vi "RF Sweep.vi"() -> ()   [LabVIEW 2012]
uses:
  <vilib>/DAQmx/read.llb/DAQmx Read (Counter U32 1Chan 1Samp).vi
  <vilib>/Utility/file.llb/Write To Spreadsheet File (DBL).vi
  <vilib>/DAQmx/miscellaneous.llb/DAQmx Fill In Error Info.vi
  <vilib>/DAQmx/create/channels.llb/DAQmx Create Channel (CO-Pulse Generation-Ticks).vi
  <vilib>/DAQmx/configure/timing.llb/DAQmx Timing (Implicit).vi
  <vilib>/DAQmx/create/channels.llb/DAQmx Create Channel (CI-Count Edges).vi
  <vilib>/DAQmx/configure/timing.llb/DAQmx Timing (Sample Clock).vi
  <resource>/objmgr/daqmx.rc
panel:
  in  "Time Target (s)":dbl=1.0
  out "freq":dbl
  out "diff":dbl
  out "loop":i32
  in  "file path (dialog if empty)":path
  out "Z Position 2":dbl
  out "Y Position 2":dbl
  out "X Position 2":dbl
  in  "CW for tracking":bool
  in  "Y Parameters":T1={"Number of Y Steps"=200, "Max Y (V)"=2.0, "Min Y (V)"=-2.0}
  in  "X":T2={"Number of X Steps"=200, "Max X (V)"=2.0, "Min X (V)"=-2.0}
  in  "Z Position":dbl
  in  "Y Position":dbl
  in  "X Position":dbl
  in  "Z-track?":bool
  out "XY Graph":cluster{"Y":dbl[], "Y":dbl[]}[](graph)
  in  "Freq Max":dbl=485493835.2340852
  in  "Freq  Step":dbl=485493835.2340852
  in  "Freq Min":dbl=485493835.2340852
  in  "power":dbl
  in  "Measure N Loops":i32
  in  "stop":bool
  out "no pi":u32
  out "pi":u32
  in  "Path to spinapi.dll":path=path "C:/SpinCore/SpinAPI/dll/spinapi64.dll"
  in  "Pulse offset":dbl
  in  "Tau":dbl
  in  "RF Pulse":dbl
  in  "Rabi Freq":dbl
  in  "MW Delay":dbl
  in  "APD signal width":dbl=5e-07
  in  "Signal Delay":dbl=6e-07
  in  "AOM Rest time":dbl=1e-06
  in  "AOM Pulse length":dbl=2.5e-06
  in  "N Loop":i32=10000
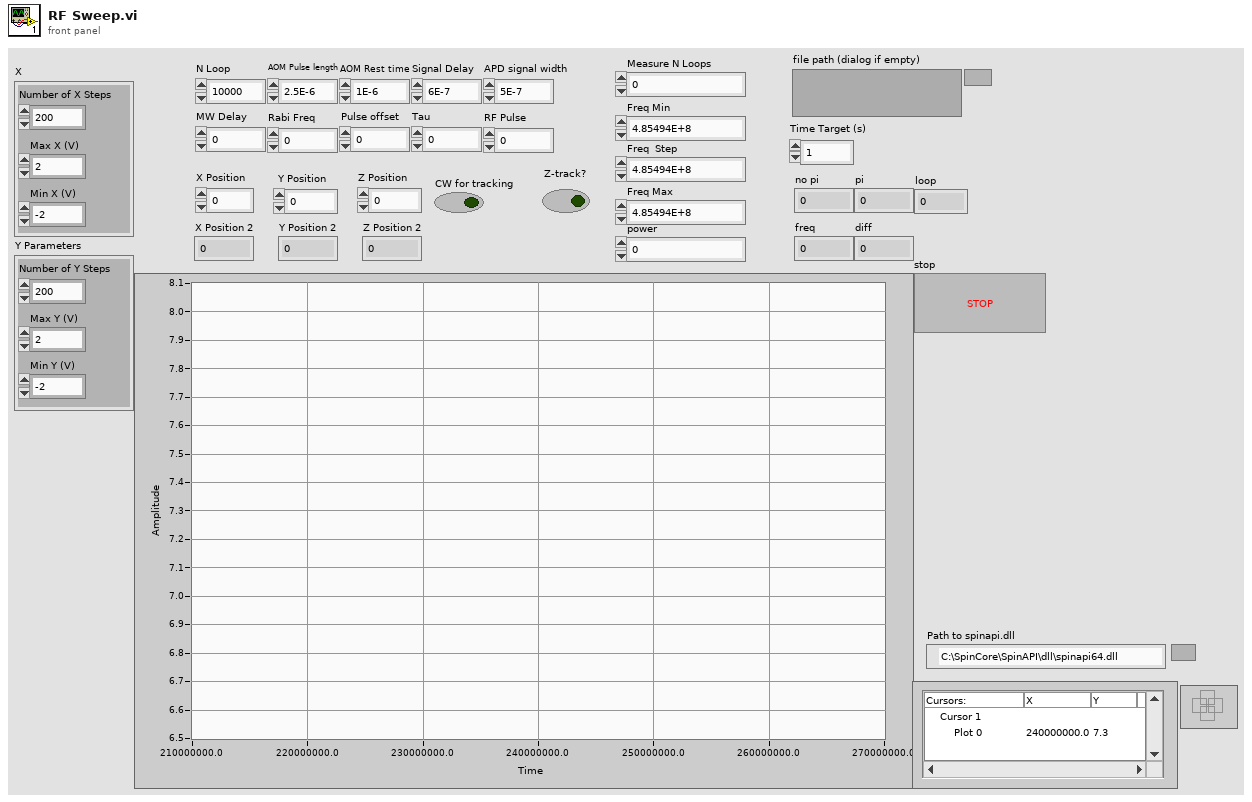
[diagram p1: front panel]
types:
  T1 = cluster{"Number of Y Steps":i32, "Max Y (V)":dbl, "Min Y (V)":dbl}
  T2 = cluster{"Number of X Steps":i32, "Max X (V)":dbl, "Min X (V)":dbl}
  T3 = enum16{"Pulse Program", "Frequency Registers", "TX Phase Registers", "RX Phase Registers"}
  T4 = cluster{"Instruct Data":i32, "Op Code":i32, "Flags":bool[], "Comments":string, "Time (s)":dbl}[]
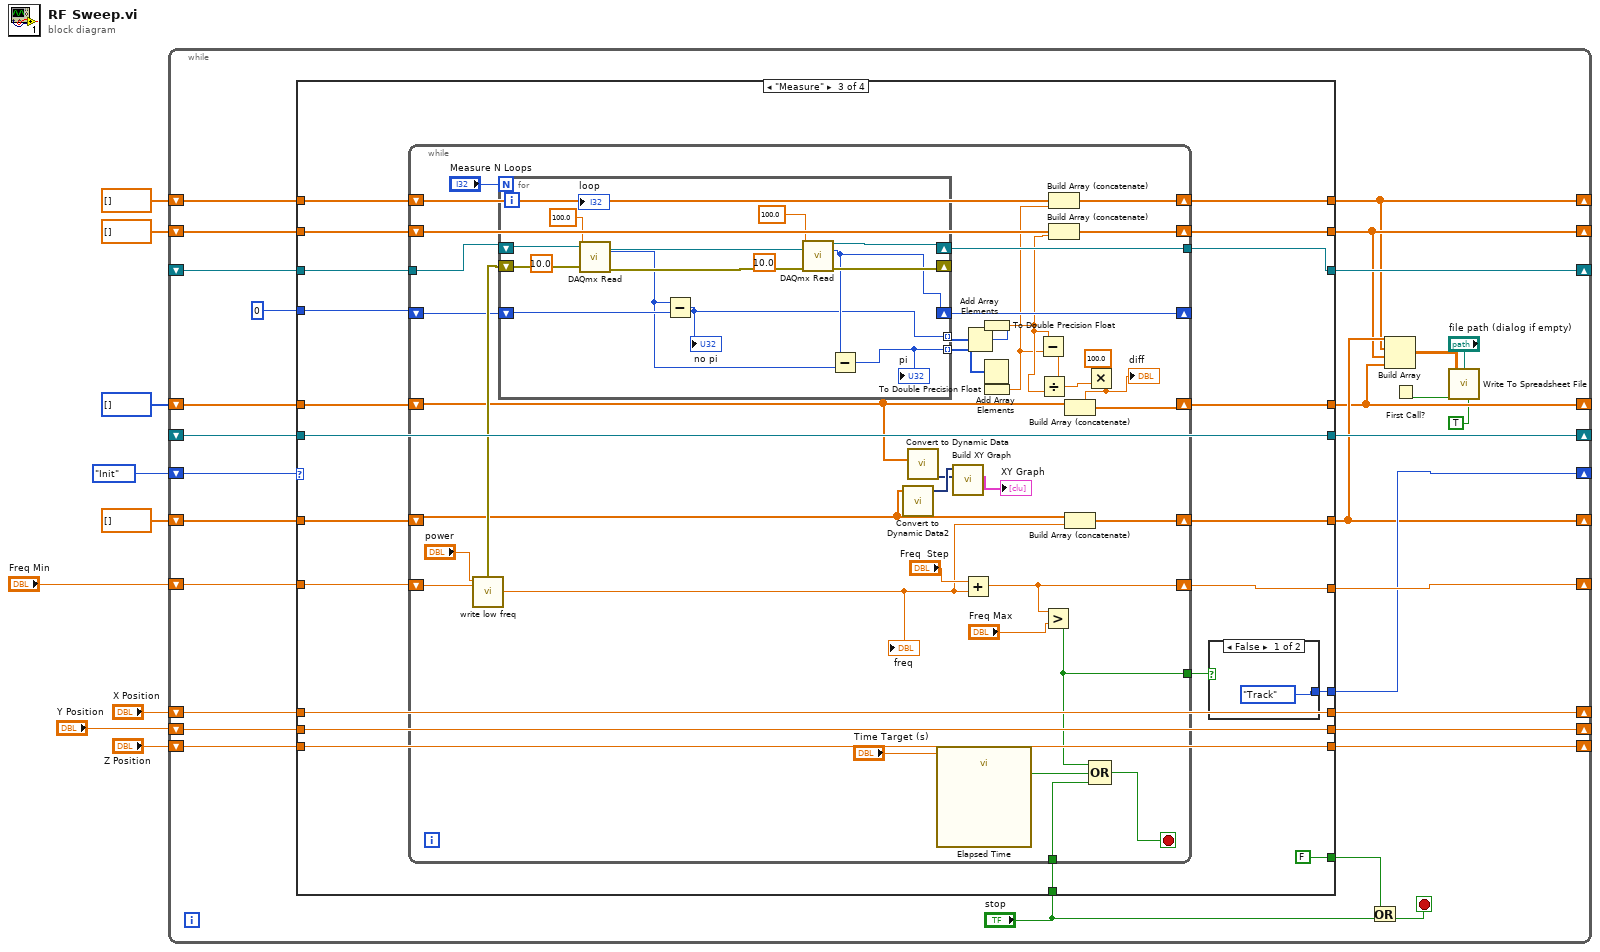
[diagram p0: block diagram]
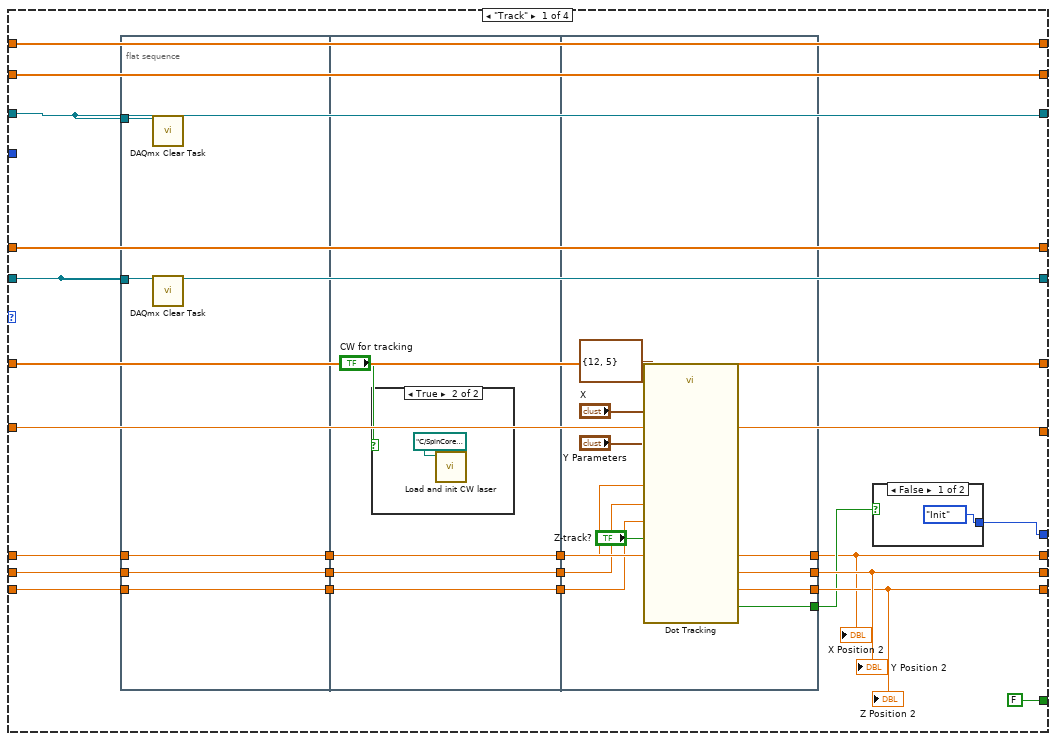
[diagram p2: hidden frame]
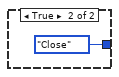
[diagram p3: hidden frame]
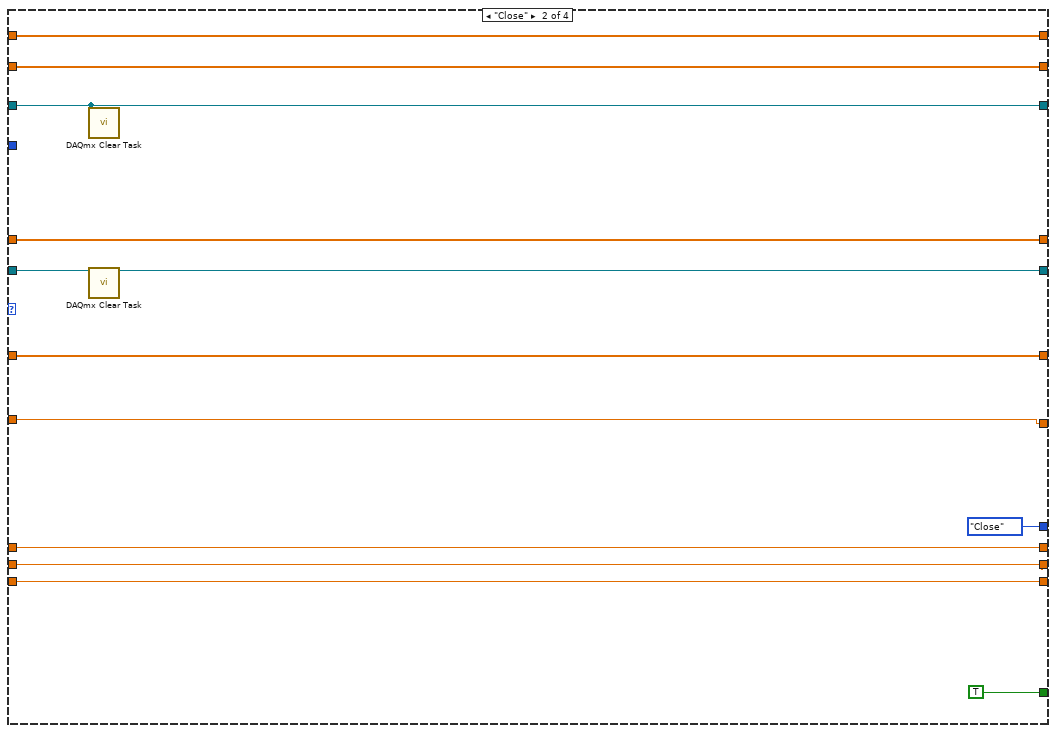
[diagram p5: hidden frame]
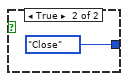
[diagram p6: hidden frame]
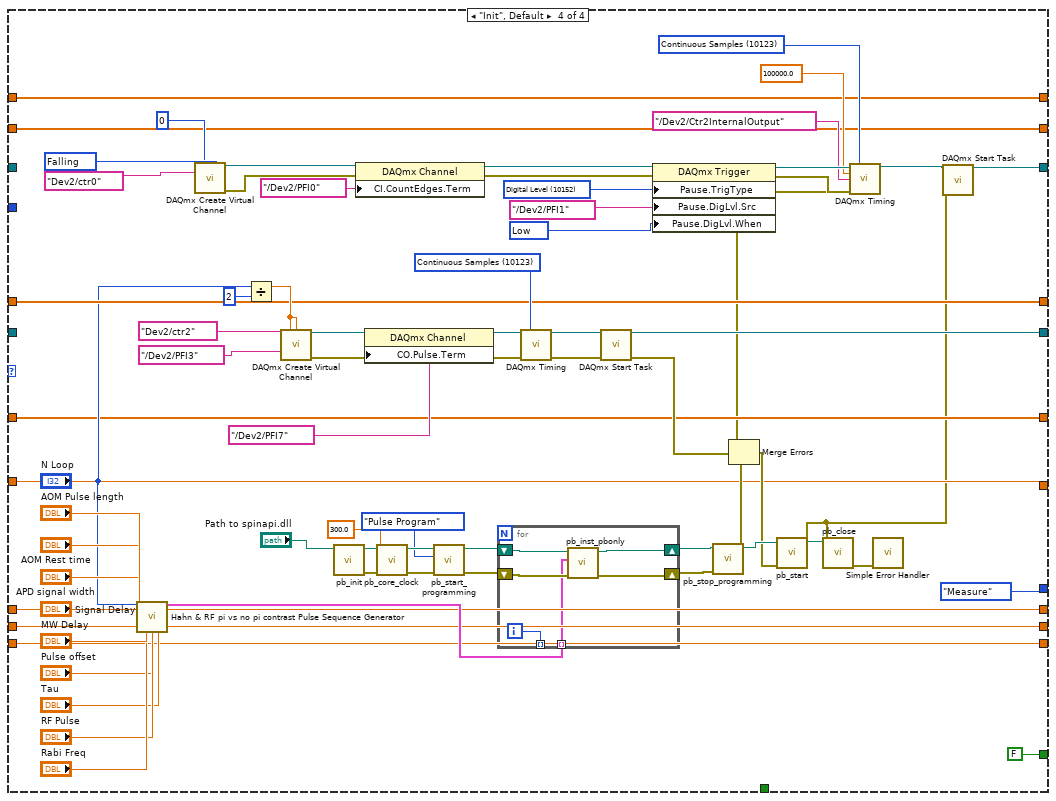
[diagram p7: hidden frame]
diagram:
  n1 = while {
    shift-right: [w31] -> _
    shift-left: enum16{"Init", "Track", "Measure", "Close", ""}."Init" -> [w39]
    shift-right: [w38] -> _
    shift-left: _ -> [w24]
    shift-right: [w37] -> _
    shift-left: _ -> [w25]
    shift-right: [w34] -> _
    shift-left: "Freq Min" -> [w35]
    shift-right: [w16] -> _
    shift-left: u32[] [] -> [w33]
    shift-right: [w17] -> _
    shift-left: dbl[] [] -> [w32]
    shift-right: [w30] -> _
    shift-left: "X Position" -> [w21]
    shift-right: [w29] -> _
    shift-left: "Y Position" -> [w27]
    shift-right: [w28] -> _
    shift-left: "Z Position" -> [w26]
    shift-right: [w10] -> _
    shift-left: dbl[] [] -> [w19]
    shift-right: [w15] -> _
    shift-left: dbl[] [] -> [w18]
    stop <- w23 stop-if-true
    n2 = case shown="\"Measure\"" w39 {
      tunnel: [w43 w95 w105 w185] -> w38
      tunnel: [w42 w94 w106 w184] -> w37
      tunnel: "stop" -> [_ _ w116 _]
      tunnel: w35 -> [w52 w92 w115 w182]
      tunnel: [w52 w92 w114 w182] -> w34
      tunnel: w33 -> [w53 w93 w113 w181]
      tunnel: w32 -> [w47 w87 w112 w176]
      tunnel: [w53 w93 w111 w181] -> w16
      tunnel: [w47 w87 w102 w176] -> w17
      tunnel: [w51 enum16{"Init", "Track", "Measure", "Close", ""}."Close" w109 enum16{"Init", "Track", "Measure", "Close", ""}."Measure"] -> w31
      tunnel: [w48 w86 w101 w175] -> w30
      tunnel: [w60 w91 w104 w179] -> w29
      tunnel: [w59 w90 w103 w178] -> w28
      tunnel: w27 -> [w56 w91 w104 w179]
      tunnel: w26 -> [w54 w90 w103 w178]
      tunnel: w25 -> [w42 w94 w107 _]
      tunnel: w24 -> [w43 w95 w105 _]
      tunnel: [FALSE TRUE FALSE FALSE] -> w22
      tunnel: w21 -> [w48 w86 w101 w175]
      tunnel: u32 0 ("data") -> [_ _ w100 _]
      tunnel: [w41 w85 w99 w173] -> w10
      tunnel: [w40 w84 w98 w172] -> w15
      tunnel: w19 -> [w41 w85 w97 w173]
      tunnel: w18 -> [w40 w84 w96 w172]
      frame "Track" {
        n3 = flat-sequence {
          tunnel: w54 -> [w65]
          tunnel: w56 -> [w66]
          tunnel: w48 -> [w67]
          tunnel: [w67] -> w46
          tunnel: [w66] -> w45
          tunnel: [w65] -> w44
          tunnel: w43 -> [w64]
          tunnel: w42 -> [w63]
          tunnel: [w71] -> w58
          tunnel: [w70] -> w57
          tunnel: [w69] -> w55
          tunnel: w46 -> [w71]
          tunnel: w45 -> [w70]
          tunnel: w44 -> [w69]
          tunnel: [w83] -> _
          tunnel: [w82] -> w60
          tunnel: [w81] -> w59
          tunnel: w58 -> [w80]
          tunnel: w57 -> [w79]
          tunnel: w55 -> [w78]
          tunnel: [w73] -> w50
          frame #0 {
            n4 = call <vilib>:"DAQmx Clear Task.vi"("task in"=w63) -> ()  [unwired: 14 in, 1 out]
            n5 = call <vilib>:"DAQmx Clear Task.vi"("task in"=w64) -> ()  [unwired: 14 in, 1 out]
          }
          frame #1 {
            n6 = case shown="True" "CW for tracking" {
              frame False {
              }
              frame True {
                n7 = call "Load and init CW laser.vi"("path in"=path "C:/SpinCore/SpinAPI/dll/spinapi64.dll") -> ()  [unwired: 11 in]
              }
            }
          }
          frame #2 {
            n8 = call "Dot Tracking.vi"("X"="X", "Y Parameters"="Y Parameters", "RS232 settings"=cluster{"Portnumber":i32, "Baudrate":u16} {"Portnumber"=12, "Baudrate"=5}, "X Pos"=w80, "Y pos"=w79, "Z Pos"=w78, "Z-track?"="Z-track?") -> ("X Position"=w83:dbl, "Y Position"=w82:dbl, "Z Position"=w81:dbl, "Gave up?"=w73:bool)  [unwired: 2 in, 3 out]
          }
        }
        n9 = case shown="False" w50 {
          tunnel: [enum16{"Init", "Track", "Measure", "Close", ""}."Init" enum16{"Init", "Track", "Measure", "Close", ""}."Close"] -> w51
          frame False {
          }
          frame True {
          }
        }
        "X Position 2" <- w48
        "Y Position 2" <- w60
        "Z Position 2" <- w59
      }
      frame "Close" {
        n10 = call <vilib>:"DAQmx Clear Task.vi"("task in"=w94) -> ()  [unwired: 14 in, 1 out]
        n11 = call <vilib>:"DAQmx Clear Task.vi"("task in"=w95) -> ()  [unwired: 14 in, 1 out]
      }
      frame "Measure" {
        n12 = while {
          tunnel: w116 -> [w149]
          shift-right: [w147] -> w114
          shift-left: w115 -> [w141]
          shift-right: [w143] -> w111
          shift-left: w113 -> [w129]
          shift-right: [w142] -> w102
          shift-left: w112 -> [w138]
          tunnel: [w137] -> w110
          tunnel: w107 -> [w136]
          tunnel: [w135] -> w106
          shift-right: [w128] -> _
          shift-left: w100 -> [w127]
          shift-right: [w126] -> w99
          shift-left: w97 -> [w124]
          shift-right: [w125] -> w98
          shift-left: w96 -> [w123]
          stop <- w150 stop-if-true
          n13 = call "write low freq.vi"("Freq"=w141, "power"="power") -> ("error out"=w140:errorcluster)  [unwired: 9 in]
          n14 = for {
            N: "Measure N Loops" -> [_]
            shift-right: [w165] -> w135
            shift-left: w136 -> [w169]
            shift-right: [w164] -> w128
            shift-left: w127 -> [w168]
            shift-right: [w166] -> _
            shift-left: w140 -> [w167]
            tunnel: [w163] -> w155 mode=indexing
            tunnel: [w162] -> w154 mode=indexing
            i -> [w156]
            (unwired) 10.0 ("timeout")
            (unwired) 10.0 ("timeout")
            n15 = call-poly <vilib>:"DAQmx Read.vi"("task/channels in"=w169, "timeout"=100.0, "error in"=w167) -> ("task out"=w160:refnum<k21>, "data"=w157:u32, "error out"=w159:errorcluster)  [unwired: 10 in]
            n16 = Subtract(x=w157, y=w168) -> (x-y=w163:u32)
            "no pi" <- w163
            n17 = call-poly <vilib>:"DAQmx Read.vi"("task/channels in"=w160, "timeout"=100.0, "error in"=w159) -> ("task out"=w165:refnum<k21>, "data"=w164:u32, "error out"=w166:errorcluster)  [unwired: 10 in]
            n18 = Subtract(x=w164, y=w157) -> (x-y=w162:u32)
            "pi" <- w162
            "loop" <- w156
          }
          n19 = call "Convert to Dynamic Data2"("Array"=w138) -> ("Dynamic Data Type"=w133:dynamicdata)  [unwired: 3 in]
          n20 = call "Convert to Dynamic Data"("Array"=w129) -> ("Dynamic Data Type"=w132:dynamicdata)  [unwired: 3 in]
          n21 = call "Elapsed Time"("Time Target (s)"="Time Target (s)") -> ("Time has Elapsed"=w151:bool)  [unwired: 11 in, 7 out]
          n22 = call "Build XY Graph"("Y Input"=w132, "X Input"=w133) -> ("XY Graph"=→"XY Graph":cluster{"Y":dbl[], "Y":dbl[]}[])  [unwired: 3 in, 6 out]
          n23 = Add(x="Freq  Step", y=w141) -> (x+y=w147:dbl)
          n24 = Add Array Elements(numeric array=w155) -> (sum=w145:u32)
          n25 = Add Array Elements(numeric array=w154) -> (sum=w144:u32)
          n26 = To Double Precision Float(number=w145) -> (double precision float=w122:dbl)
          n27 = To Double Precision Float(number=w144) -> (double precision float=w121:dbl)
          n28 = Subtract(x=w122, y=w121) -> (x-y=w120:dbl)
          n29 = Divide(x=w120, y=w122) -> (x/y=w134:dbl)
          n30 = Greater?(x=w147, y="Freq Max") -> (0:w137:bool)
          n31 = Build Array (concatenate)(w124, w121) -> (w126:dbl[])
          n32 = Build Array (concatenate)(w123, w122) -> (w125:dbl[])
          n33 = Build Array (concatenate)(w138, w141) -> (w142:dbl[])
          n34 = Multiply(x=100.0, y=w134) -> (x*y=w119:dbl)
          "diff" <- w119
          n35 = Build Array (concatenate)(w129, w119) -> (w143:dbl[])
          n36 = Compound Arithmetic op=OR(w137, w151, w149) -> (w150:bool)
          "freq" <- w141
        }
        n37 = case shown="False" w110 {
          tunnel: [enum16{"Init", "Track", "Measure", "Close", ""}."Track" enum16{"Init", "Track", "Measure", "Close", ""}."Close"] -> w109
          frame False {
          }
          frame True {
          }
        }
      }
      frame "Init", Default {
        w193 = 10123 items=["Finite Samples"=10178, "Continuous Samples"=10123, "Hardware Timed Single Point"=12522] ("sample mode")
        w213 = 10214 items=["High"=10192, "Low"=10214] ("Pause.DigLvl.When")
        w215 = 10152 items=["Analog Level"=10101, "Analog Window"=10103, "Digital Level"=10152, "Digital Pattern"=10398, "None"=10230] ("Pause.TrigType")
        w202 = 10123 items=["Finite Samples"=10178, "Continuous Samples"=10123, "Hardware Timed Single Point"=12522] ("sample mode")
        w189 = 10171 items=["Rising"=10280, "Falling"=10171] ("edge")
        n38 = call "Hahn & RF pi vs no pi contrast Pulse Sequence Generator.vi"("N Loop"="N Loop", "Rabi Frequency"="Rabi Freq", "RF Pulse"="RF Pulse", "Tau"="Tau", "AOM Pulse length"="AOM Pulse length", "AOM Rest time"="AOM Rest time", "Signal Delay"="Signal Delay", "APD signal width"="APD signal width", "MW Delay"="MW Delay", "Pulse offset"="Pulse offset") -> ("Pulse Sequence"=w216:T4)  [unwired: 5 in]
        n39 = call-poly <vilib>:"DAQmx Create Virtual Channel.vi"("initial count"=u32 0, "edge"=w189, "counter"=tag "Dev2/ctr0") -> ("task out"=w211:refnum<k21>, "error out"=w208:errorcluster)  [unwired: 6 in, 5 out]
        n40 = Divide(x="N Loop", y=2) -> (x/y=w199:dbl)
        n41 = call-poly <vilib>:"DAQmx Create Virtual Channel.vi"("high ticks"=w199, "low ticks"=w199, "counter"=tag "Dev2/ctr2", "source of ticks"=tag "/Dev2/PFI3" ("source")) -> ("task out"=w197:refnum<k21>, "error out"=w195:errorcluster)  [unwired: 10 in]
        n42 = call "pb_init.vi"("path in"="Path to spinapi.dll") -> ("error out"=w222:errorcluster, "path out"=w220:path)  [unwired: 3 in, 6 out]
        n43 = property class="DAQmx Channel"(reference=w211, error in=w208, "CI.CountEdges.Term"=tag "/Dev2/PFI0") -> (reference out=w212:refnum<k21>, error out=w210:errorcluster)
        n44 = property class="DAQmx Channel"(reference=w197, "CO.Pulse.Term"=tag "/Dev2/PFI7") -> (reference out=w192:refnum<k21>)  [unwired: 1 in, 1 out]
        n45 = call "pb_core_clock.vi"("error in (no error)"=w222, "clock_freq (MHz)"=300.0, "path in"=w220) -> ("error out"=w223:errorcluster, "path out"=w221:path)  [unwired: 7 in]
        n46 = call "pb_start_programming.vi"("error in (no error)"=w223, "Device"=T3."Pulse Program", "path in"=w221) -> ("error out"=w226:errorcluster, "path out"=w225:path)  [unwired: 1 in, 6 out]
        n47 = for {
          shift-right: [w243] -> w227
          shift-left: w225 -> [w245]
          shift-right: [w242] -> w228
          shift-left: w226 -> [w244]
          tunnel: [w241] -> _ mode=indexing
          tunnel: w216 -> [w240] mode=indexing
          i -> [w241]
          n48 = call "pb_inst_pbonly.vi"("error in (no error)"=w244, "PB Instruction"=w240, "path in"=w245) -> ("error out"=w242:errorcluster, "path out"=w243:path)  [unwired: 2 in, 5 out]
        }
        n49 = call-poly <vilib>:"DAQmx Timing.vi"("task/channels in"=w192, "sample mode"=w193, "error in"=w195) -> ("task out"=w196:refnum<k21>, "error out"=w194:errorcluster)  [unwired: 11 in]
        n50 = call <vilib>:"DAQmx Start Task.vi"("task/channels in"=w196, "error in"=w194) -> ("task out"=w185:refnum<k21>, "error out"=w188:errorcluster)  [unwired: 12 in]
        n51 = property class="DAQmx Trigger"(reference=w212, error in=w210, "Pause.TrigType"=w215, "Pause.DigLvl.Src"=tag "/Dev2/PFI1", "Pause.DigLvl.When"=w213) -> (reference out=w207:refnum<k21>, error out=w206:errorcluster)
        n52 = call "pb_stop_programming.vi"("error in (no error)"=w228, "path in"=w227) -> ("error out"=w186:errorcluster, "path out"=w218:path)  [unwired: 1 in, 7 out]
        n53 = call-poly <vilib>:"DAQmx Timing.vi"("task/channels in"=w207, "sample mode"=w202, "rate"=100000.0, "source"=tag "/Dev2/Ctr2InternalOutput", "error in"=w206) -> ("task out"=w204:refnum<k21>, "error out"=w171:errorcluster)  [unwired: 9 in]
        n54 = Merge Errors(w171, w188, w186) -> (w187:errorcluster)
        n55 = call "pb_start.vi"("error in (no error)"=w187, "path in"=w218) -> ("error out"=w170:errorcluster, "path out"=w217:path)  [unwired: 1 in, 7 out]
        n56 = call "pb_close.vi"("error in (no error)"=w170, "path in"=w217) -> ("error out"=w230:errorcluster)  [unwired: 9 out]
        n57 = call <vilib>:"Simple Error Handler.vi"("error in (no error)"=w230) -> ()  [unwired: 1 in, 8 out]
        n58 = call <vilib>:"DAQmx Start Task.vi"("task/channels in"=w204, "error in"=w170) -> ("task out"=w184:refnum<k21>)  [unwired: 13 out]
      }
    }
    n59 = Or(x=w22, y="stop") -> (x .or. y?=w23:bool)
    n60 = Build Array(w17, w10, w15, w16) -> (w14:dbl[][])
    n61 = First Call?() -> (First Call?: T/F=w11:bool)
    n62 = call-poly <vilib>:"Write To Spreadsheet File.vi"("transpose? (no:F)"=TRUE, "append to file? (new file:F)"=w11, "2D data"=w14, "file path (dialog if empty)"="file path (dialog if empty)") -> ()  [unwired: 4 in, 1 out]
  }
